vi "IV readmethod.vi"(8 "error in (no error)":errorcluster, 11 "fname":string) -> (0 "error out":errorcluster, 2 "return type":i32, 3 "fname out":string)   [LabVIEW 2020, in "IVIUM_remdriver.lvlib"]
uses:
  IVIUM_remdriver.lvlib
  SEC Software V4.9/Dependencies/Drivers and Aux files/IVIUM/IVIUM_remdriver.dll
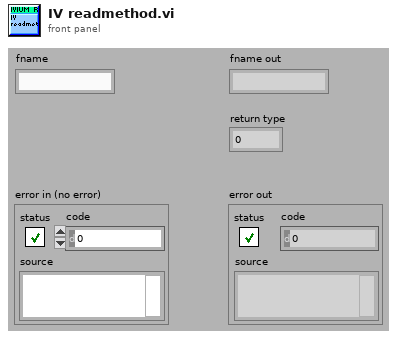
[diagram p1: front panel]
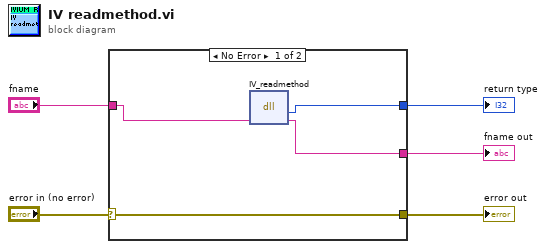
[diagram p0: block diagram]
diagram:
  n1 = case shown="No Error" "error in (no error)" {
    selector: "error in (no error)" -> [w9 w11]
    tunnel: [w9 w11] -> w4
    tunnel: [w8 _] -> w3
    tunnel: "fname" -> [w7 w10]
    tunnel: [w6 w10] -> w1
    frame No Error {
      n2 = dll-call lib="C:/Users/Benj/Desktop/SEC Software V4.9/Dependencies/Drivers and Aux files/IVIUM/IVIUM_remdriver.*" fn="IV_readmethod"("fname"=w7) -> (w8:i32, "fname"=w6:string)  [unwired: 3 in, 2 out]
    }
    frame Error {
    }
  }
  "return type" <- w3
  "fname out" <- w1
  "error out" <- w4
